vi "Untitled 1.vi"() -> ()   [LabVIEW 2020]
panel:
  in  "'":i32=1
  out "Slide 2":dbl(slide) scale=0.0..300.0
  in  "Array 2  1":dbl
  in  "Array 2   0":dbl
  out "Numeric 3":i32
  in  "Array 1   1":dbl
  in  "Array 1   0":dbl
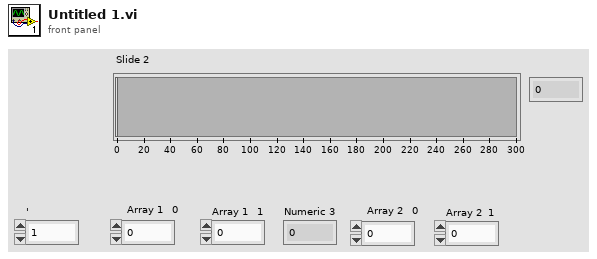
[diagram p1: front panel]
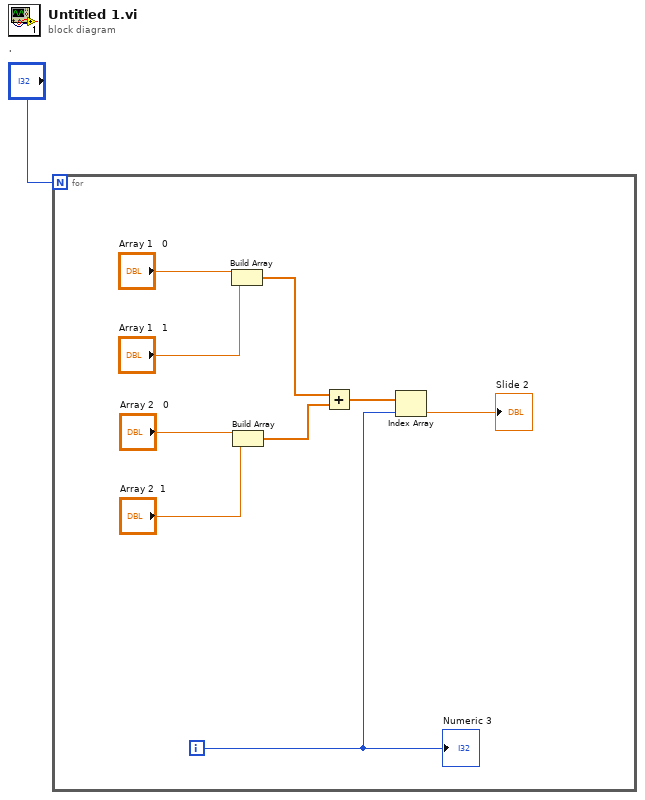
[diagram p0: block diagram]
diagram:
  n1 = for {
    N: "'" -> [_]
    i -> [w3]
    n2 = Build Array("Array 1   0", "Array 1   1") -> (w8:dbl[])
    n3 = Build Array("Array 2   0", "Array 2  1") -> (w5:dbl[])
    n4 = Add(x=w8, y=w5) -> (x+y=w4:dbl[])
    n5 = Index Array(array=w4, index=w3) -> (element=→"Slide 2":dbl)
    "Numeric 3" <- w3
  }
